vi "电流曲线.vi"(6 "Time Resolution(s) 2":dbl=0.05, 7 "0安培电流保持时间":dbl=50.0, 8 "总持续时间(s)":dbl=100.0, 10 "x的第二个值决定斜率（建议0.02）":dbl, 11 "IR":dbl=100.0) -> (2 "输出电流值":dbl[](array[numeric]))   [LabVIEW 2018]
panel:
  out "查询的y":dbl[](array[numeric]) format="%.3g"
  out "稳态电流":dbl
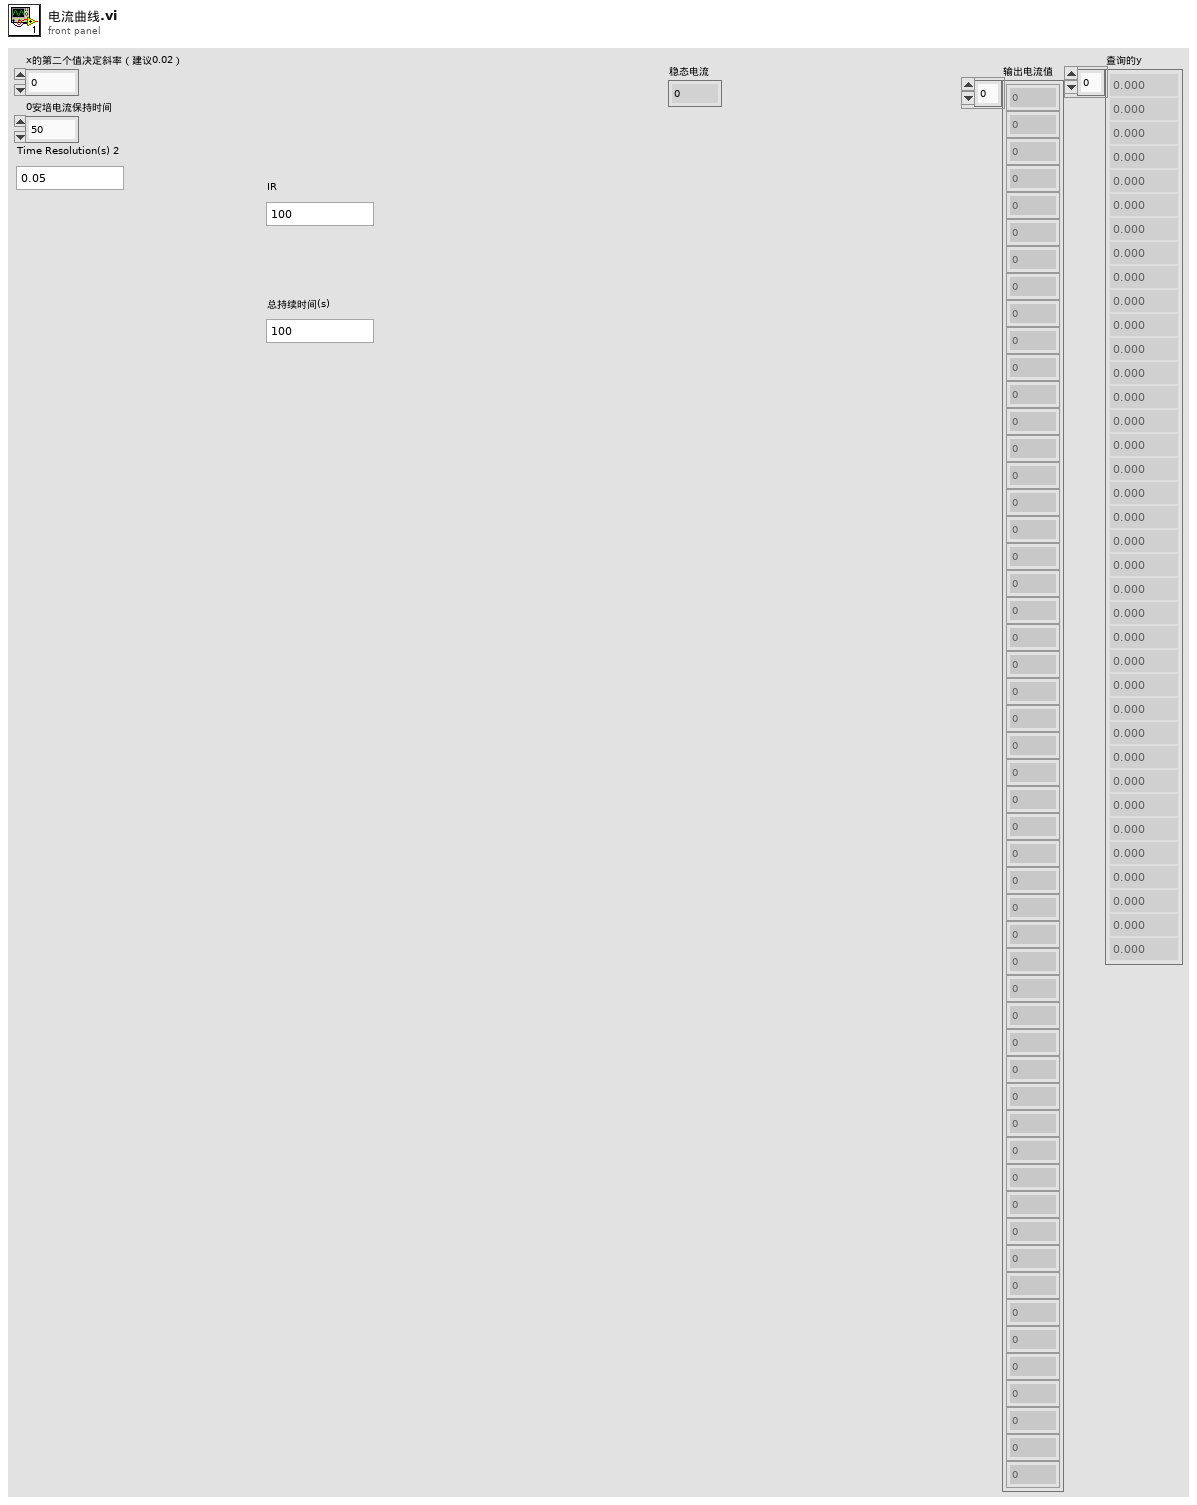
[diagram p1: front panel]
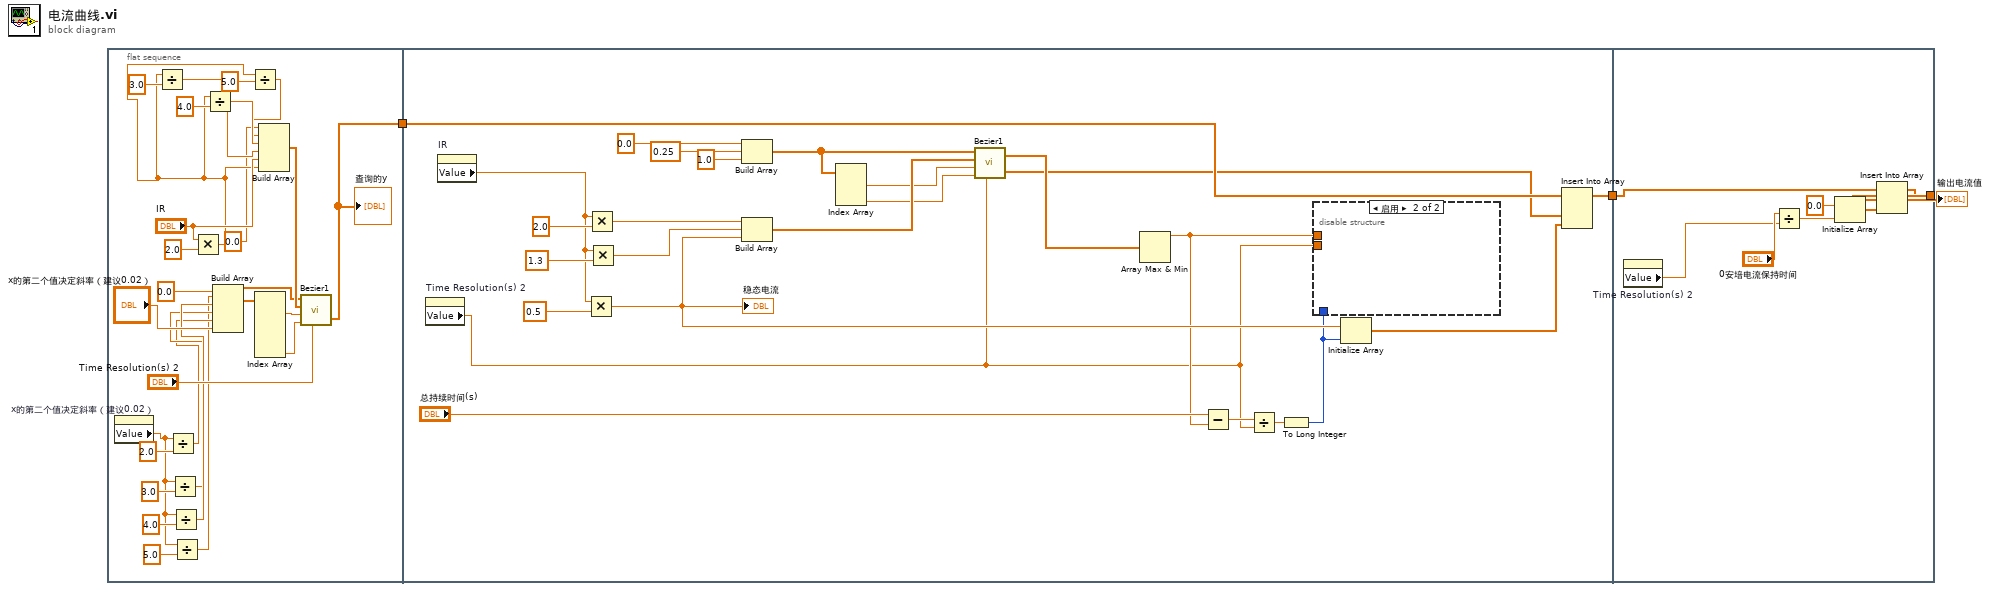
[diagram p0: block diagram]
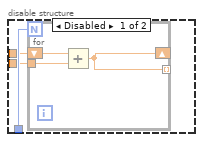
[diagram p2: hidden frame]
diagram:
  n1 = flat-sequence {
    tunnel: [w26] -> w1
    tunnel: [w55] -> w2
    tunnel: w1 -> [w35]
    tunnel: [w67] -> w3
    tunnel: w2 -> [w68]
    frame #0 {
      n2 = property on="x的第二个值决定斜率（建议0.02）" class="DigNum (严格)"() -> ("Value"=w12:dbl)  [unwired: 2 in, 2 out]
      n3 = Divide(x=w12, y=2.0) -> (x/y=w18:dbl)
      n4 = Divide(x=w12, y=3.0) -> (x/y=w19:dbl)
      n5 = Divide(x=w12, y=4.0) -> (x/y=w20:dbl)
      n6 = Divide(x=w12, y=5.0) -> (x/y=w9:dbl)
      n7 = Multiply(x="IR", y=2.0) -> (x*y=w7:dbl)
      n8 = Divide(x=w7, y=3.0) -> (x/y=w14:dbl)
      n9 = Divide(x=w7, y=4.0) -> (x/y=w15:dbl)
      n10 = Build Array(0.0 ("元素"), w9, w20, w19, w18, "x的第二个值决定斜率（建议0.02）") -> (w29:dbl[])
      n11 = Divide(x=w7, y=5.0) -> (x/y=w5:dbl)
      n12 = Index Array(array=w29) -> (element #1=w28:dbl, element #6=w4:dbl)  [unwired: 6 in, 4 out]
      n13 = Build Array(0.0 ("元素"), w5, w15, w14, "IR", w7) -> (w30:dbl[])
      n14 = call "Bezier1.vi"("d"="Time Resolution(s) 2", "y"=w4, "x"=w28, "Y"=w30, "X"=w29) -> ("查询的y"=w26:dbl[])  [unwired: 1 in, 1 out]
      "查询的y" <- w26
    }
    frame #1 {
      n15 = property on="Time Resolution(s) 2" class="DigNum (严格)"() -> ("Value"=w36:dbl)  [unwired: 2 in, 2 out]
      n16 = property on="IR" class="DigNum (严格)"() -> ("Value"=w31:dbl)  [unwired: 2 in, 2 out]
      n17 = Multiply(x=w31, y=0.5) -> (x*y=w42:dbl)
      "稳态电流" <- w42
      n18 = Multiply(x=w31, y=2.0) -> (x*y=w32:dbl)
      n19 = Multiply(x=w31, y=1.3) -> (x*y=w50:dbl)
      n20 = Build Array(0.0 ("元素"), 0.25 ("元素"), 1.0 ("元素")) -> (w45:dbl[])
      n21 = Build Array(w32, w50, w42) -> (w48:dbl[])
      n22 = Index Array(array=w45) -> (element #1=w44:dbl, element #3=w43:dbl)  [unwired: 3 in, 1 out]
      n23 = call "Bezier1.vi"("d"=w36, "y"=w43, "x"=w44, "Y"=w48, "X"=w45) -> ("查询的y"=w34:dbl[], "待查找值"=w37:dbl[])  [unwired: 1 in]
      n24 = Array Max & Min(array=w37) -> (max value=w38:dbl)  [unwired: 3 out]
      n25 = Subtract(x="总持续时间(s)", y=w38) -> (x-y=w41:dbl)
      n26 = Divide(x=w41, y=w36) -> (x/y=w40:dbl)
      n27 = To Long Integer(number=w40) -> (32bit integer=w39:i32)
      n28 = disable-structure shown="启用" {
        disable-tunnel: w39 -> [w58 _]
        disable-tunnel: w38 -> [w57 _]
        disable-tunnel: w36 -> [w56 _]
        frame Disabled {
          n29 = for {
            N: w58 -> [_]
            tunnel: w56 -> [w60]
            shift-right: [w59] -> _
            shift-left: w57 -> [w61]
            tunnel: [w59] -> _ mode=indexing
            n30 = Add(x=w61, y=w60) -> (x+y=w59:dbl)
          }
        }
        frame Enabled {
        }
      }
      n31 = Initialize Array(w42, w39) -> (w33:dbl[])
      n32 = Insert Into Array(array=w35, new element #1=w34, new element #2=w33) -> (w55:dbl[])  [unwired: 1 in]
    }
    frame #2 {
      n33 = property on="Time Resolution(s) 2" class="DigNum (严格)"() -> ("Value"=w62:dbl)  [unwired: 2 in, 2 out]
      n34 = Divide(x="0安培电流保持时间", y=w62) -> (x/y=w64:dbl)
      n35 = Initialize Array(0.0 ("元素"), w64) -> (w63:dbl[])
      n36 = Insert Into Array(array=w68, new element=w63) -> (w67:dbl[])  [unwired: 1 in]
    }
  }
  "输出电流值" <- w3
